vi "DSF.Engine.Runtime.Framework.Initialize.vi"(8 "error in (no error)":errorcluster, 9 "Device Item Ref":T1=18446744073709551615 format="%.0x", 10 "Framework Configuration":refnum<class "DSF.Shared.Configuration.Framework.lvclass">, 11 "Framework Runtime in":refnum<class "DSF.Engine.Runtime.Framework.lvclass">) -> (0 "error out":errorcluster, 3 "Framework Runtime out":refnum<class "DSF.Engine.Runtime.Framework.lvclass">)   [LabVIEW 2016, in "DSF.Engine.lvlib" / "DSF.Engine.Runtime.Framework.lvclass"]
uses:
  DSF.Engine.Runtime.Framework.lvclass
  Shared/Classes/Framework/DSF.Shared.Configuration.Framework.lvclass
  <vilib>/NI Veristand/Custom Device API/Custom Device Item Ref.ctl
  DSF.Engine.Runtime.Framework.lvclass/DSF.Engine.Runtime.Framework.ctl
  Shared/Classes/Framework/DSF.Shared.Configuration.Framework.lvclass/DSF.Shared.Configuration.Framework.ctl
  Cache/DSF.Engine.Memory.Cache.Framework.lvclass/DSF.Engine.Memory.Cache.Framework.ctl
  Cache/DSF.Engine.Memory.Cache.Plugin.lvclass/DSF.Engine.Memory.Cache.Plugin.ctl
  Cache/DSF.Engine.Memory.Cache.Transfer Group.lvclass/DSF.Engine.Memory.Cache.Transfer Group.ctl
  Cache/DSF.Engine.Memory.Cache.Transfer.lvclass/DSF.Engine.Memory.Cache.Transfer.ctl
  Shared/Classes/Transfer/DSF.Shared.Configuration.Transfer.lvclass/DSF.Shared.Configuration.Transfer.ctl
  Hardware/DSF.Engine.Hardware Info.lvclass/DSF.Engine.Hardware Info.ctl
  Hardware/DSF.Engine.Hardware Info.CPU.lvclass/DSF.Engine.Hardware Info.CPU.ctl
  Sequencer/DSF.Engine.Sequencer Bundle.lvclass/DSF.Engine.Sequencer Bundle.ctl
  Plugin/DSF.Engine.Runtime.Plugin.lvclass/DSF.Engine.Runtime.Plugin.ctl
  Runtime/DSF.Engine.Runtime.lvclass/DSF.Engine.Runtime.ctl
  Sequencer/DSF.Engine.Sequencer.lvclass/DSF.Engine.Sequencer.ctl
  DSF.Engine.Runtime.Framework.Get Configuration.vi
  DSF.Engine.Runtime.Framework.Set Framework Cache.vi
  Cache/DSF.Engine.Memory.Cache.Framework.Initialize.vi
  DSF.Engine.Runtime.Framework.Get Device Ref.vi
  Cache/DSF.Engine.Memory.Cache.Framework.Create.vi
  DSF.Engine.Runtime.Framework.Get Framework Cache.vi
  DSF.Engine.Runtime.Framework.Set Builder Manager.vi
  DSF.Engine.Runtime.Framework.Get Hardware Info.vi
  Hardware/DSF.Engine.Hardware Info.Get CPU.vi
  Hardware/DSF.Engine.Hardware Info.CPU.Get Core Count.vi
  DSF.Engine.Runtime.Framework.Set Plugin Runtimes.vi
  DSF.Engine.Runtime.Framework.Get Plugin Runtimes.vi
  Sequencer/DSF.Engine.Sequencer.Create.vi
  DSF.Engine.Runtime.Framework.Set Sequencer.vi
  Cache/DSF.Engine.Memory.Cache.Plugin.Initialize.vi
  Cache/DSF.Engine.Memory.Cache.Framework.Get Plugin Caches.vi
  Cache/DSF.Engine.Memory.Cache.Framework.Set Plugin Caches.vi
  Cache/DSF.Engine.Memory.Cache.Framework.Set Framework Configuration.vi
  Shared/Classes/Framework/DSF.Shared.Configuration.Framework.Get Plugin Configurations.vi
  Runtime/DSF.Engine.Runtime.Get Timing.vi
  Sequencer/DSF.Engine.Sequencer Bundle.Set Iteration.vi
  Sequencer/DSF.Engine.Sequencer Bundle.Set Plugin Timing.vi
  Sequencer/DSF.Engine.Sequencer Bundle.Set Transfer Group Timings.vi
  Plugin/DSF.Engine.Runtime.Plugin.Get Cache.vi
  Cache/DSF.Engine.Memory.Cache.Plugin.Get Transfer Group Caches.vi
  Cache/DSF.Engine.Memory.Cache.Transfer Group.Get Timing.vi
  Sequencer/DSF.Engine.Sequencer.Set Plugin Bundles.vi
  Cache/DSF.Engine.Memory.Cache.Transfer Group.Initialize.vi
  Cache/DSF.Engine.Memory.Cache.Plugin.Set Transfer Group Caches.vi
  Cache/DSF.Engine.Memory.Cache.Transfer Group.Set Transfer Caches.vi
  Cache/DSF.Engine.Memory.Cache.Transfer.Initialize.vi
  Cache/DSF.Engine.Memory.Cache.Transfer Group.Get Transfer Caches.vi
  Cache/DSF.Engine.Memory.Cache.Transfer.Initialize Buffer.vi
  Cache/DSF.Engine.Memory.Cache.Transfer.Initialize Channels Pointer.vi
  Shared/Classes/Transfer/DSF.Shared.Configuration.Transfer.Required Buffer Size.vi
  Cache/DSF.Engine.Memory.Cache.Transfer.Set Buffer.vi
  Cache/DSF.Engine.Memory.Cache.Transfer.Get Configuration.vi
  Cache/DSF.Engine.Memory.Cache.Transfer.Set VS Channels Pointer.vi
  Pointer/DSF.Engine.Memory.Pointer.VS Channels.New.vi
  Shared/Classes/Transfer/DSF.Shared.Configuration.Transfer.Get Block Descriptors.vi
  Shared/Classes/Transfer/DSF.Shared.Configuration.Transfer.Get Channel Count.vi
  Shared/Classes/Transfer/DSF.Shared.Configuration.Transfer.Get Access Mode.vi
  Shared/VIs/DSF.Shared.Data Type.Sizeof.1D.vi
  Pointer/DSF.Engine.Memory.Pointer.VS Channels.Data Ref to Pointer.vi
  Shared/Classes/Transfer/DSF.Shared.Configuration.Transfer.Get Channel Descriptors.vi
  Shared/Classes/Transfer/DSF.Shared.Configuration.Transfer.Get Direction.vi
  Shared/VIs/DSF.Shared.Data Type.Sizeof.vi
  Pointer/DSF.Engine.Memory.Pointer.VS Channels.lvclass
  C:/Git/Sourcetree/DSF/Source/Submodules/Memory/Source/Classes/External/Memory.Pointer.External.lvclass
  Plugin/DSF.Engine.Runtime.Plugin.lvclass
  C:/Git/Sourcetree/DSF/Source/Engine/Classes/Runtime/DSF.Engine.Runtime.lvclass
  BuilderManager/DSF.Engine.Execution.BuilderManager.New.vi
  Submodules/Memory/Source/Classes/External/Memory.Pointer.External.Encapsulate.vi
  <vilib>/NI Veristand/Custom Device API/Global Data Refs.vi
  <vilib>/NI Veristand/Custom Device API/NI VeriStand - Get Channel Data Reference.vi
  Buffer/DSF.Engine.Memory.Buffer.New.vi
  Sequencer/DSF.Engine.Sequencer Bundle.lvclass
  Sequencer/DSF.Engine.Sequencer.lvclass
  Cache/DSF.Engine.Memory.Cache.Framework.lvclass
  Cache/DSF.Engine.Memory.Cache.Plugin.lvclass
  <vilib>/NI Veristand/Custom Device API/Custom Device API.lvlib
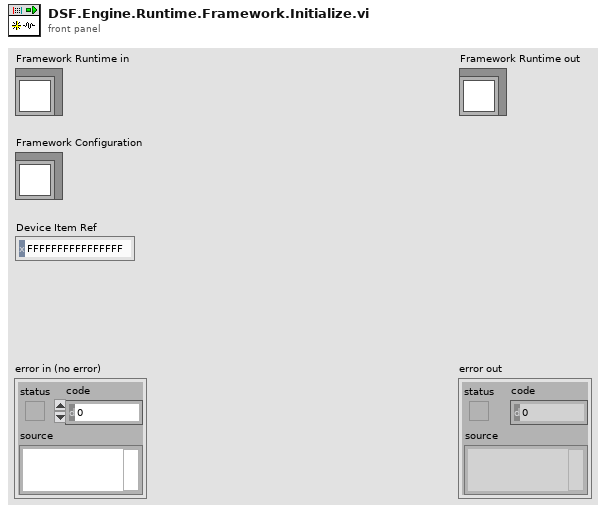
[diagram p1: front panel]
types:
  T1 = typedef "Custom Device API.lvlib/Custom Device Item Ref.ctl" = u64
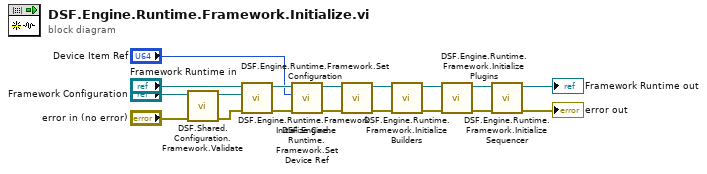
[diagram p0: block diagram]
diagram:
  n1 = call "DSF.Shared.Configuration.Framework.Validate.vi"("error in (no error)"="error in (no error)", "Framework Configuration in"="Framework Configuration") -> ("error out"=w15:errorcluster, "Framework Configuration out"=w14:refnum<class "DSF.Shared.Configuration.Framework.lvclass">)  [unwired: 8 in]
  n2 = call "DSF.Engine.Runtime.Framework.Set Configuration.vi"("error in (no error)"=w15, "Framework Configuration"=w14, "Framework Runtime in"="Framework Runtime in") -> ("error out"=w12:errorcluster, "Framework Runtime out"=w13:refnum<class "DSF.Engine.Runtime.Framework.lvclass">)  [unwired: 7 in]
  n3 = call "DSF.Engine.Runtime.Framework.Set Device Ref.vi"("error in (no error)"=w12, "Device Item Ref"="Device Item Ref", "Framework Runtime in"=w13) -> ("error out"=w10:errorcluster, "Framework Runtime out"=w11:refnum<class "DSF.Engine.Runtime.Framework.lvclass">)  [unwired: 7 in]
  n4 = call "DSF.Engine.Runtime.Framework.Initialize Cache.vi"("error in (no error)"=w10, "Framework Runtime in"=w11) -> ("error out"=w7:errorcluster, "Framework Runtime out"=w8:refnum<class "DSF.Engine.Runtime.Framework.lvclass">)  [unwired: 8 in]
  n5 = call "DSF.Engine.Runtime.Framework.Initialize Builders.vi"("error in (no error)"=w7, "Framework Runtime in"=w8) -> ("error out"=w5:errorcluster, "Framework Runtime out"=w6:refnum<class "DSF.Engine.Runtime.Framework.lvclass">)  [unwired: 8 in]
  n6 = call "DSF.Engine.Runtime.Framework.Initialize Plugins.vi"("error in (no error)"=w5, "Framework Runtime in"=w6) -> ("error out"=w3:errorcluster, "Framework Runtime out"=w4:refnum<class "DSF.Engine.Runtime.Framework.lvclass">)  [unwired: 8 in]
  n7 = call "DSF.Engine.Runtime.Framework.Initialize Sequencer.vi"("error in (no error)"=w3, "Framework Runtime in"=w4) -> ("error out"=→"error out":errorcluster, "Framework Runtime out"=→"Framework Runtime out":refnum<class "DSF.Engine.Runtime.Framework.lvclass">)  [unwired: 8 in]
